vi "construct.vi"(8 "error in (no error)":errorcluster, 9 "configuration name":string, 10 "load config file?":bool=TRUE, 11 "ScanModeDL090923Scaffold in":refnum<class "ImagingModeDL090923Scaffold.lvclass">) -> (0 "error out":errorcluster, 3 "ScanModeDL090923Scaffold out":refnum<class "ImagingModeDL090923Scaffold.lvclass">)   [LabVIEW 2010, in "ImagingModeDL090923Scaffold.lvclass"]
uses:
  ImagingModeDL090923Scaffold.lvclass
  GenericImagingMode/GenericImagingMode/GenericImagingMode.lvclass
  Trajectory/GenericTrajectory/GenericTrajectory/GenericTrajectory.lvclass
  ImagingModeDL090923Scaffold.lvclass/ImagingModeDL090923Scaffold.ctl
  common/classes/ErrorController/ErrorController/class_data.vi
  Adapter/GenericAdapter/GenericAdapter/GenericAdapter.lvclass
  common/classes/GenericComponent/GenericComponent/GenericComponent.lvclass
  common/classes/ErrorController/ErrorController/ErrorController.lvclass
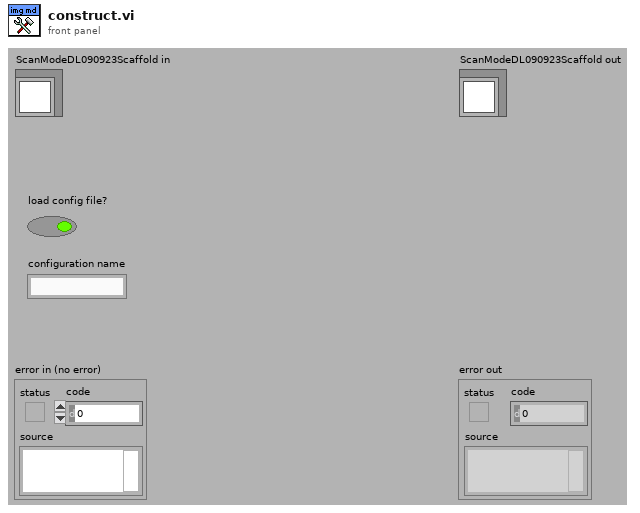
[diagram p1: front panel]
types:
  T1 = typedef "plugin_specification.ctl" = cluster{"class path":string, "configuration":string, "label":string, "settings name":string}
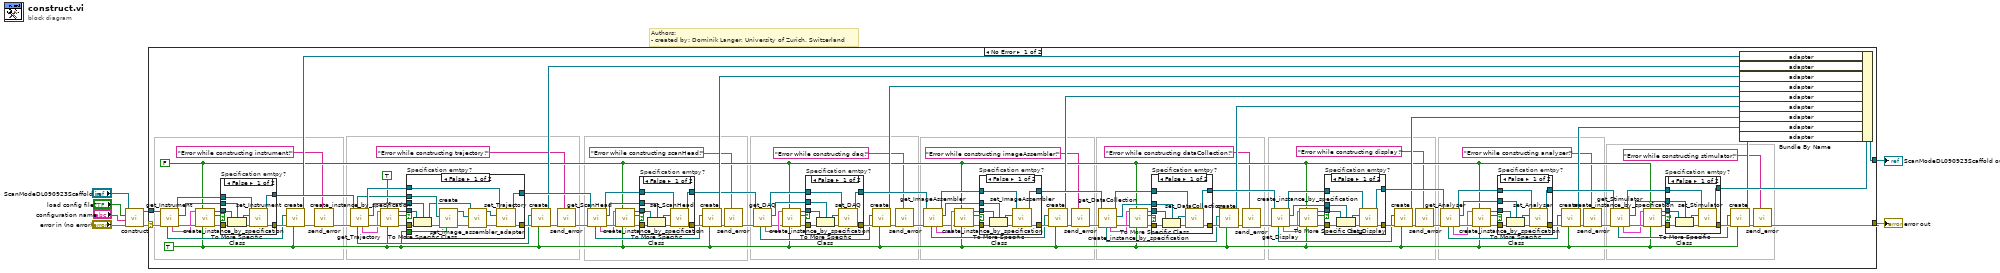
[diagram p0: block diagram]
diagram:
  # "Authors: \n- created by: Dominik Langer, University of Zurich, Switzerland"
  n1 = call-parent "construct.vi"("error in (no error)"="error in (no error)", "configuration name"="configuration name", "load config file?"="load config file?", "GenericPlugin in"="ScanModeDL090923Scaffold in") -> ("error out"=w4:errorcluster, "GenericPlugin out"=w3:refnum<class "ImagingModeDL090923Scaffold.lvclass">)  [unwired: 6 in]
  n2 = case shown="No Error" w4 {
    selector: w4 -> [w125 w238]
    tunnel: w3 -> [w112 w239]
    tunnel: [w12 w238] -> w2
    tunnel: [w62 w239] -> w1
    frame No Error {
      w36 = FALSE ("call constructor?")
      w47 = TRUE
      n3 = call-dynamic "get_Instrument.vi"("error in (no error)"=w125, "ScanModeDL090923Scaffold in"=w112) -> ("error out"=w124:errorcluster, "Instrument"=w122:refnum<class "GenericInstrument.lvclass">, "ScanModeDL090923Scaffold out"=w116:refnum<class "ImagingModeDL090923Scaffold.lvclass">, "Instrument specification"=w123:T1, "adapter path"=w80:path)  [unwired: 4 in, 1 out]
      n4 = call "create_instance_by_specification.vi"("be tolerant against empty specification?"=w47, "call constructor?"=w36, "error in (no error)"=w124, "component specification"=w123) -> ("error out"=w127:errorcluster, "empty specification!"=w46:bool, "GenericPlugin out"=w126:refnum<class "GenericComponent.lvclass">)  [unwired: 5 in]
      n5 = case "Specification emtpy?" shown="False" w46 {
        tunnel: w127 -> [w234 w236]
        tunnel: w126 -> [w233 _]
        tunnel: w122 -> [w231 _]
        tunnel: [w230 w237] -> w117
        tunnel: w116 -> [w229 w237]
        tunnel: [w228 w236] -> w81
        frame False {
          n6 = To More Specific Class(target class=w231, reference=w233, error in=w234) -> (specific class reference=w232:refnum<class "GenericInstrument.lvclass">, error out=w235:errorcluster)
          n7 = call-dynamic "set_Instrument.vi"("error in (no error)"=w235, "GenericInstrument.lvclass"=w232, "ScanModeDL090923Scaffold in"=w229) -> ("error out"=w228:errorcluster, "ScanModeDL090923Scaffold out"=w230:refnum<class "ImagingModeDL090923Scaffold.lvclass">)  [unwired: 7 in]
        }
        frame True {
        }
      }
      n8 = call "create.vi"("be tolerant against empty path?"=w47, "error in (no error)"=w81, "class path"=w80) -> ("error out"=w35:errorcluster, "GenericAdapter out"=w52:refnum<class "GenericAdapter.lvclass">)  [unwired: 7 in]
      n9 = call "send_error.vi"("additional message"="Error while constructing instrument!", "error in (no error)"=w35) -> ("error out"=w34:errorcluster)  [unwired: 9 in]
      n10 = call-dynamic "get_Trajectory.vi"("error in (no error)"=w34, "ScanModeDL090923Scaffold in"=w117) -> ("error out"=w121:errorcluster, "Trajectory"=w119:refnum<class "GenericTrajectory.lvclass">, "ScanModeDL090923Scaffold out"=w49:refnum<class "ImagingModeDL090923Scaffold.lvclass">, "specification"=w120:T1, "adapter path"=w77:path, "Trajectory-to-ImageAssembler adapter path"=w48:path)  [unwired: 2 in, 2 out]
      n11 = call "create_instance_by_specification.vi"("be tolerant against empty specification?"=w47, "call constructor?"=TRUE, "error in (no error)"=w121, "component specification"=w120) -> ("error out"=w129:errorcluster, "empty specification!"=w45:bool, "GenericPlugin out"=w128:refnum<class "GenericComponent.lvclass">)  [unwired: 5 in]
      n12 = case "Specification emtpy?" shown="False" w45 {
        tunnel: w129 -> [w213 w227]
        tunnel: w128 -> [w212 _]
        tunnel: w119 -> [w225 _]
        tunnel: [w224 w227] -> w79
        tunnel: [w223 w226] -> w78
        tunnel: w49 -> [w222 w226]
        tunnel: w48 -> [w220 _]
        tunnel: w47 -> [w218 _]
        frame False {
          n13 = To More Specific Class(target class=w225, reference=w212, error in=w213) -> (specific class reference=w214:refnum<class "GenericTrajectory.lvclass">, error out=w217:errorcluster)
          n14 = call "create.vi"("be tolerant against empty path?"=w218, "error in (no error)"=w217, "class path"=w220) -> ("error out"=w216:errorcluster, "GenericAdapter out"=w215:refnum<class "GenericAdapter.lvclass">)  [unwired: 7 in]
          n15 = call-dynamic "set_image_assembler_adapter.vi"("error in (no error)"=w216, "GenericAdapter.lvclass"=w215, "GenericTrajectory in"=w214) -> ("error out"=w221:errorcluster, "GenericTrajectory out"=w219:refnum<class "GenericTrajectory.lvclass">)  [unwired: 7 in]
          n16 = call-dynamic "set_Trajectory.vi"("error in (no error)"=w221, "GenericTrajectory.lvclass"=w219, "ScanModeDL090923Scaffold in"=w222) -> ("error out"=w224:errorcluster, "ScanModeDL090923Scaffold out"=w223:refnum<class "ImagingModeDL090923Scaffold.lvclass">)  [unwired: 7 in]
        }
        frame True {
        }
      }
      n17 = call "create.vi"("be tolerant against empty path?"=w47, "error in (no error)"=w79, "class path"=w77) -> ("error out"=w32:errorcluster, "GenericAdapter out"=w53:refnum<class "GenericAdapter.lvclass">)  [unwired: 7 in]
      n18 = call "send_error.vi"("additional message"="Error while constructing trajectory!", "error in (no error)"=w32) -> ("error out"=w31:errorcluster)  [unwired: 9 in]
      n19 = call-dynamic "get_ScanHead.vi"("error in (no error)"=w31, "ScanModeDL090923Scaffold in"=w78) -> ("error out"=w118:errorcluster, "ScanHead"=w113:refnum<class "GenericScanHead.lvclass">, "ScanModeDL090923Scaffold out"=w115:refnum<class "ImagingModeDL090923Scaffold.lvclass">, "ScanHead specification"=w114:T1, "adapter path"=w75:path)  [unwired: 4 in, 1 out]
      n20 = call "create_instance_by_specification.vi"("be tolerant against empty specification?"=w47, "call constructor?"=w36, "error in (no error)"=w118, "component specification"=w114) -> ("error out"=w132:errorcluster, "empty specification!"=w44:bool, "GenericPlugin out"=w135:refnum<class "GenericComponent.lvclass">)  [unwired: 5 in]
      n21 = case "Specification emtpy?" shown="False" w44 {
        tunnel: w135 -> [w209 _]
        tunnel: w132 -> [w208 w210]
        tunnel: w115 -> [w206 w211]
        tunnel: w113 -> [w205 _]
        tunnel: [w203 w210] -> w76
        tunnel: [w202 w211] -> w51
        frame False {
          n22 = To More Specific Class(target class=w205, reference=w209, error in=w208) -> (specific class reference=w204:refnum<class "GenericScanHead.lvclass">, error out=w207:errorcluster)
          n23 = call-dynamic "set_ScanHead.vi"("error in (no error)"=w207, "GenericScanHead.lvclass"=w204, "ScanModeDL090923Scaffold in"=w206) -> ("error out"=w203:errorcluster, "ScanModeDL090923Scaffold out"=w202:refnum<class "ImagingModeDL090923Scaffold.lvclass">)  [unwired: 7 in]
        }
        frame True {
        }
      }
      n24 = call "create.vi"("be tolerant against empty path?"=w47, "error in (no error)"=w76, "class path"=w75) -> ("error out"=w29:errorcluster, "GenericAdapter out"=w54:refnum<class "GenericAdapter.lvclass">)  [unwired: 7 in]
      n25 = call "send_error.vi"("additional message"="Error while constructing scanHead!", "error in (no error)"=w29) -> ("error out"=w28:errorcluster)  [unwired: 9 in]
      n26 = call-dynamic "get_DAQ.vi"("error in (no error)"=w28, "ScanModeDL090923Scaffold in"=w51) -> ("error out"=w110:errorcluster, "DAQ"=w109:refnum<class "GenericDAQ.lvclass">, "ScanModeDL090923Scaffold out"=w50:refnum<class "ImagingModeDL090923Scaffold.lvclass">, "DAQ specification"=w111:T1, "adapter path"=w73:path)  [unwired: 4 in, 1 out]
      n27 = call "create_instance_by_specification.vi"("be tolerant against empty specification?"=w47, "call constructor?"=w36, "error in (no error)"=w110, "component specification"=w111) -> ("error out"=w141:errorcluster, "empty specification!"=w43:bool, "GenericPlugin out"=w139:refnum<class "GenericComponent.lvclass">)  [unwired: 5 in]
      n28 = case "Specification emtpy?" shown="False" w43 {
        tunnel: w141 -> [w199 w201]
        tunnel: w139 -> [w198 _]
        tunnel: w109 -> [w196 _]
        tunnel: [w194 w200] -> w103
        tunnel: [w193 w201] -> w74
        tunnel: w50 -> [w192 w200]
        frame False {
          n29 = To More Specific Class(target class=w196, reference=w198, error in=w199) -> (specific class reference=w195:refnum<class "GenericDAQ.lvclass">, error out=w197:errorcluster)
          n30 = call-dynamic "set_DAQ.vi"("error in (no error)"=w197, "GenericDAQ.lvclass"=w195, "ScanModeDL090923Scaffold in"=w192) -> ("error out"=w193:errorcluster, "ScanModeDL090923Scaffold out"=w194:refnum<class "ImagingModeDL090923Scaffold.lvclass">)  [unwired: 7 in]
        }
        frame True {
        }
      }
      n31 = call "create.vi"("be tolerant against empty path?"=w47, "error in (no error)"=w74, "class path"=w73) -> ("error out"=w26:errorcluster, "GenericAdapter out"=w55:refnum<class "GenericAdapter.lvclass">)  [unwired: 7 in]
      n32 = call "send_error.vi"("additional message"="Error while constructing daq!", "error in (no error)"=w26) -> ("error out"=w25:errorcluster)  [unwired: 9 in]
      n33 = call-dynamic "get_ImageAssembler.vi"("error in (no error)"=w25, "ScanModeDL090923Scaffold in"=w103) -> ("error out"=w100:errorcluster, "ImageAssembler"=w99:refnum<class "GenericImageAssembler.lvclass">, "ScanModeDL090923Scaffold out"=w102:refnum<class "ImagingModeDL090923Scaffold.lvclass">, "ImageAssembler specification"=w101:T1, "adapter path"=w71:path)  [unwired: 4 in, 1 out]
      n34 = call "create_instance_by_specification.vi"("be tolerant against empty specification?"=w47, "call constructor?"=w36, "error in (no error)"=w100, "component specification"=w101) -> ("error out"=w140:errorcluster, "empty specification!"=w42:bool, "GenericPlugin out"=w136:refnum<class "GenericComponent.lvclass">)  [unwired: 5 in]
      n35 = case "Specification emtpy?" shown="False" w42 {
        tunnel: w140 -> [w189 w190]
        tunnel: w136 -> [w188 _]
        tunnel: w102 -> [w185 w191]
        tunnel: w99 -> [w184 _]
        tunnel: [w183 w191] -> w89
        tunnel: [w182 w190] -> w72
        frame False {
          n36 = To More Specific Class(target class=w184, reference=w188, error in=w189) -> (specific class reference=w186:refnum<class "GenericImageAssembler.lvclass">, error out=w187:errorcluster)
          n37 = call-dynamic "set_ImageAssembler.vi"("error in (no error)"=w187, "GenericImageAssembler.lvclass"=w186, "ScanModeDL090923Scaffold in"=w185) -> ("error out"=w182:errorcluster, "ScanModeDL090923Scaffold out"=w183:refnum<class "ImagingModeDL090923Scaffold.lvclass">)  [unwired: 7 in]
        }
        frame True {
        }
      }
      n38 = call "create.vi"("be tolerant against empty path?"=w47, "error in (no error)"=w72, "class path"=w71) -> ("error out"=w23:errorcluster, "GenericAdapter out"=w56:refnum<class "GenericAdapter.lvclass">)  [unwired: 7 in]
      n39 = call "send_error.vi"("additional message"="Error while constructing imageAssembler!", "error in (no error)"=w23) -> ("error out"=w22:errorcluster)  [unwired: 9 in]
      n40 = call-dynamic "get_DataCollection.vi"("error in (no error)"=w22, "ScanModeDL090923Scaffold in"=w89) -> ("error out"=w92:errorcluster, "DataCollection"=w90:refnum<class "GenericDataCollection.lvclass">, "ScanModeDL090923Scaffold out"=w87:refnum<class "ImagingModeDL090923Scaffold.lvclass">, "DataCollection specification"=w91:T1, "adapter path"=w69:path)  [unwired: 4 in, 1 out]
      n41 = call "create_instance_by_specification.vi"("be tolerant against empty specification?"=w47, "call constructor?"=w36, "error in (no error)"=w92, "component specification"=w91) -> ("error out"=w93:errorcluster, "empty specification!"=w41:bool, "GenericPlugin out"=w94:refnum<class "GenericComponent.lvclass">)  [unwired: 5 in]
      n42 = case "Specification emtpy?" shown="False" w41 {
        tunnel: w94 -> [w179 _]
        tunnel: w93 -> [w178 w180]
        tunnel: w90 -> [w175 _]
        tunnel: [w174 w181] -> w88
        tunnel: w87 -> [w173 w181]
        tunnel: [w172 w180] -> w70
        frame False {
          n43 = To More Specific Class(target class=w175, reference=w179, error in=w178) -> (specific class reference=w176:refnum<class "GenericDataCollection.lvclass">, error out=w177:errorcluster)
          n44 = call-dynamic "set_DataCollection.vi"("error in (no error)"=w177, "GenericDataCollection.lvclass"=w176, "ScanModeDL090923Scaffold in"=w173) -> ("error out"=w172:errorcluster, "ScanModeDL090923Scaffold out"=w174:refnum<class "ImagingModeDL090923Scaffold.lvclass">)  [unwired: 7 in]
        }
        frame True {
        }
      }
      n45 = call "create.vi"("be tolerant against empty path?"=w47, "error in (no error)"=w70, "class path"=w69) -> ("error out"=w20:errorcluster, "GenericAdapter out"=w57:refnum<class "GenericAdapter.lvclass">)  [unwired: 7 in]
      n46 = call "send_error.vi"("additional message"="Error while constructing dataCollection!", "error in (no error)"=w20) -> ("error out"=w19:errorcluster)  [unwired: 9 in]
      n47 = call-dynamic "get_Display.vi"("error in (no error)"=w19, "ScanModeDL090923Scaffold in"=w88) -> ("error out"=w98:errorcluster, "Display"=w96:refnum<class "GenericDisplay.lvclass">, "ScanModeDL090923Scaffold out"=w97:refnum<class "ImagingModeDL090923Scaffold.lvclass">, "Display specification"=w95:T1, "adapter path"=w67:path)  [unwired: 4 in, 1 out]
      n48 = call "create_instance_by_specification.vi"("be tolerant against empty specification?"=w47, "call constructor?"=w36, "error in (no error)"=w98, "component specification"=w95) -> ("error out"=w138:errorcluster, "empty specification!"=w40:bool, "GenericPlugin out"=w137:refnum<class "GenericComponent.lvclass">)  [unwired: 5 in]
      n49 = case "Specification emtpy?" shown="False" w40 {
        tunnel: w138 -> [w169 w170]
        tunnel: w137 -> [w168 _]
        tunnel: w97 -> [w165 w171]
        tunnel: w96 -> [w164 _]
        tunnel: [w163 w171] -> w86
        tunnel: [w162 w170] -> w68
        frame False {
          n50 = To More Specific Class(target class=w164, reference=w168, error in=w169) -> (specific class reference=w166:refnum<class "GenericDisplay.lvclass">, error out=w167:errorcluster)
          n51 = call-dynamic "set_Display.vi"("error in (no error)"=w167, "GenericDisplay.lvclass"=w166, "ScanModeDL090923Scaffold in"=w165) -> ("error out"=w162:errorcluster, "ScanModeDL090923Scaffold out"=w163:refnum<class "ImagingModeDL090923Scaffold.lvclass">)  [unwired: 7 in]
        }
        frame True {
        }
      }
      n52 = call "create.vi"("be tolerant against empty path?"=w47, "error in (no error)"=w68, "class path"=w67) -> ("error out"=w15:errorcluster, "GenericAdapter out"=w58:refnum<class "GenericAdapter.lvclass">)  [unwired: 7 in]
      n53 = call "send_error.vi"("additional message"="Error while constructing display!", "error in (no error)"=w15) -> ("error out"=w14:errorcluster)  [unwired: 9 in]
      n54 = call-dynamic "get_Analyser.vi"("error in (no error)"=w14, "ScanModeDL090923Scaffold in"=w86) -> ("error out"=w84:errorcluster, "Analyser"=w82:refnum<class "GenericAnalyser.lvclass">, "ScanModeDL090923Scaffold out"=w85:refnum<class "ImagingModeDL090923Scaffold.lvclass">, "Analyser specification"=w83:T1, "adapter path"=w63:path)  [unwired: 4 in, 1 out]
      n55 = call "create_instance_by_specification.vi"("be tolerant against empty specification?"=w47, "call constructor?"=w36, "error in (no error)"=w84, "component specification"=w83) -> ("error out"=w133:errorcluster, "empty specification!"=w39:bool, "GenericPlugin out"=w134:refnum<class "GenericComponent.lvclass">)  [unwired: 5 in]
      n56 = case "Specification emtpy?" shown="False" w39 {
        tunnel: w134 -> [w159 _]
        tunnel: w133 -> [w158 w161]
        tunnel: [w156 w160] -> w107
        tunnel: w85 -> [w154 w160]
        tunnel: w82 -> [w153 _]
        tunnel: [w152 w161] -> w64
        frame False {
          n57 = To More Specific Class(target class=w153, reference=w159, error in=w158) -> (specific class reference=w155:refnum<class "GenericAnalyser.lvclass">, error out=w157:errorcluster)
          n58 = call-dynamic "set_Analyser.vi"("error in (no error)"=w157, "Analyser"=w155, "ScanModeDL090923Scaffold in"=w154) -> ("error out"=w152:errorcluster, "ScanModeDL090923Scaffold out"=w156:refnum<class "ImagingModeDL090923Scaffold.lvclass">)  [unwired: 7 in]
        }
        frame True {
        }
      }
      n59 = call "create.vi"("be tolerant against empty path?"=w47, "error in (no error)"=w64, "class path"=w63) -> ("error out"=w16:errorcluster, "GenericAdapter out"=w59:refnum<class "GenericAdapter.lvclass">)  [unwired: 7 in]
      n60 = call "send_error.vi"("additional message"="Error while constructing analyser!", "error in (no error)"=w16) -> ("error out"=w13:errorcluster)  [unwired: 9 in]
      n61 = call-dynamic "get_Stimulator.vi"("error in (no error)"=w13, "ScanModeDL090923Scaffold in"=w107) -> ("error out"=w108:errorcluster, "Stimulator"=w104:refnum<class "GenericStimulator.lvclass">, "ScanModeDL090923Scaffold out"=w106:refnum<class "ImagingModeDL090923Scaffold.lvclass">, "Stimulator specification"=w105:T1, "adapter path"=w65:path)  [unwired: 4 in, 1 out]
      n62 = call "create_instance_by_specification.vi"("be tolerant against empty specification?"=w47, "call constructor?"=w36, "error in (no error)"=w108, "component specification"=w105) -> ("error out"=w130:errorcluster, "empty specification!"=w38:bool, "GenericPlugin out"=w131:refnum<class "GenericComponent.lvclass">)  [unwired: 5 in]
      n63 = case "Specification emtpy?" shown="False" w38 {
        tunnel: w131 -> [w149 _]
        tunnel: w130 -> [w148 w150]
        tunnel: w106 -> [w146 w151]
        tunnel: w104 -> [w145 _]
        tunnel: [w143 w150] -> w66
        tunnel: [w142 w151] -> w61
        frame False {
          n64 = To More Specific Class(target class=w145, reference=w149, error in=w148) -> (specific class reference=w144:refnum<class "GenericStimulator.lvclass">, error out=w147:errorcluster)
          n65 = call-dynamic "set_Stimulator.vi"("error in (no error)"=w147, "GenericStimulator.lvclass"=w144, "ScanModeDL090923Scaffold in"=w146) -> ("error out"=w143:errorcluster, "ScanModeDL090923Scaffold out"=w142:refnum<class "ImagingModeDL090923Scaffold.lvclass">)  [unwired: 7 in]
        }
        frame True {
        }
      }
      n66 = call "create.vi"("be tolerant against empty path?"=w47, "error in (no error)"=w66, "class path"=w65) -> ("error out"=w17:errorcluster, "GenericAdapter out"=w60:refnum<class "GenericAdapter.lvclass">)  [unwired: 7 in]
      n67 = Bundle By Name(cluster=w61, "adapter"=w52, "adapter"=w53, "adapter"=w54, "adapter"=w55, "adapter"=w56, "adapter"=w57, "adapter"=w58, "adapter"=w59, "adapter"=w60) -> (w62:refnum<class "ImagingModeDL090923Scaffold.lvclass">)
      n68 = call "send_error.vi"("additional message"="Error while constructing stimulator!", "error in (no error)"=w17) -> ("error out"=w12:errorcluster)  [unwired: 9 in]
    }
    frame Error {
    }
  }
  "error out" <- w2
  "ScanModeDL090923Scaffold out" <- w1
